vi "Actor Core.vi"(8 "error in":errorcluster, 11 "State in":refnum<class "Keypad.lvclass">) -> (0 "error out":errorcluster, 3 "Actor out":refnum<class "Actor.lvclass">)   [LabVIEW 2020, in "Keypad.lvlib" / "Keypad.lvclass"]
doc: "(<B>Filename</B>: Actor Framework.lvlib:Actor.lvclass:Actor Core.vi)\n\nThis override invokes Entry.vi on the initial state, prior to calling the parent Actor Core. Adding this behavior to Actor Core (instead of an override of Pre Launch Init.vi) allows the initial state to launch a nested actor as part of its entry behavior.\n\nReceives messages to the actor, reacts to them, and initiates any error handling that may shut the actor down.\n\nDescendant classes may override this VI to append parallel tasks for the actor to complete while it handles messages. Overrides use the Call Parent Method node."
uses:
  Keypad.lvclass
  <vilib>/ni/Actors/State Actor/State Actor/State Actor.lvclass
  <vilib>/ActorFramework/Actor/Actor.lvclass
  <vilib>/ActorFramework/Stop Msg/Stop Msg.lvclass
  Keypad Messages/Key Pressed Msg/Key Pressed Msg.lvclass
  Keypad Messages/Set NumLock Msg/Set NumLock Msg.lvclass
  Type Def - Entry Keypad Cluster.ctl
  Type Def - Cursor Display.ctl
panel:
  out "Locked?":bool
  in  "Num Lock":bool
  out "Cursor":T1
  in  "Keypad Cluster":T2
  out "Text":string
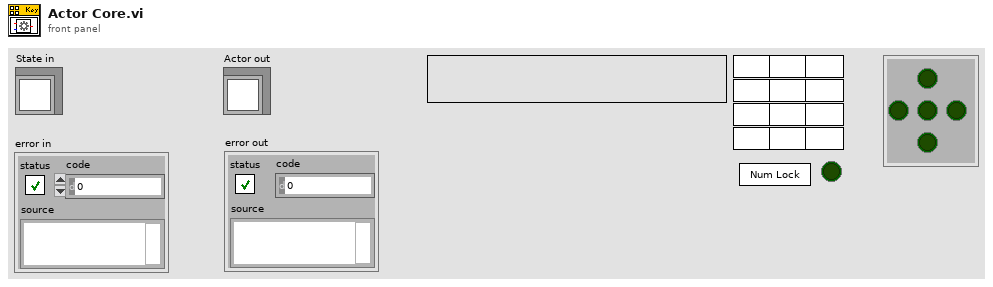
[diagram p1: front panel]
types:
  T1 = typedef "Type Def - Cursor Display.ctl" = cluster{"Up":bool, "Left":bool, "Ctr":bool, "Right":bool, "Down":bool}
  T2 = typedef "Type Def - Entry Keypad Cluster.ctl" = cluster{"K 0":bool, "K 1":bool, "K 2":bool, "K 3":bool, "K 4":bool, "K 5":bool, "K 6":bool, "K 7":bool, "K 8":bool, "K 9":bool, "K C":bool, "K E":bool}
  T3 = cluster{"Stop":refnum<user-event>, "Labels":refnum<user-event>, "Text":refnum<user-event>, "Cursor":refnum<user-event>, "NumLock":refnum<user-event>}
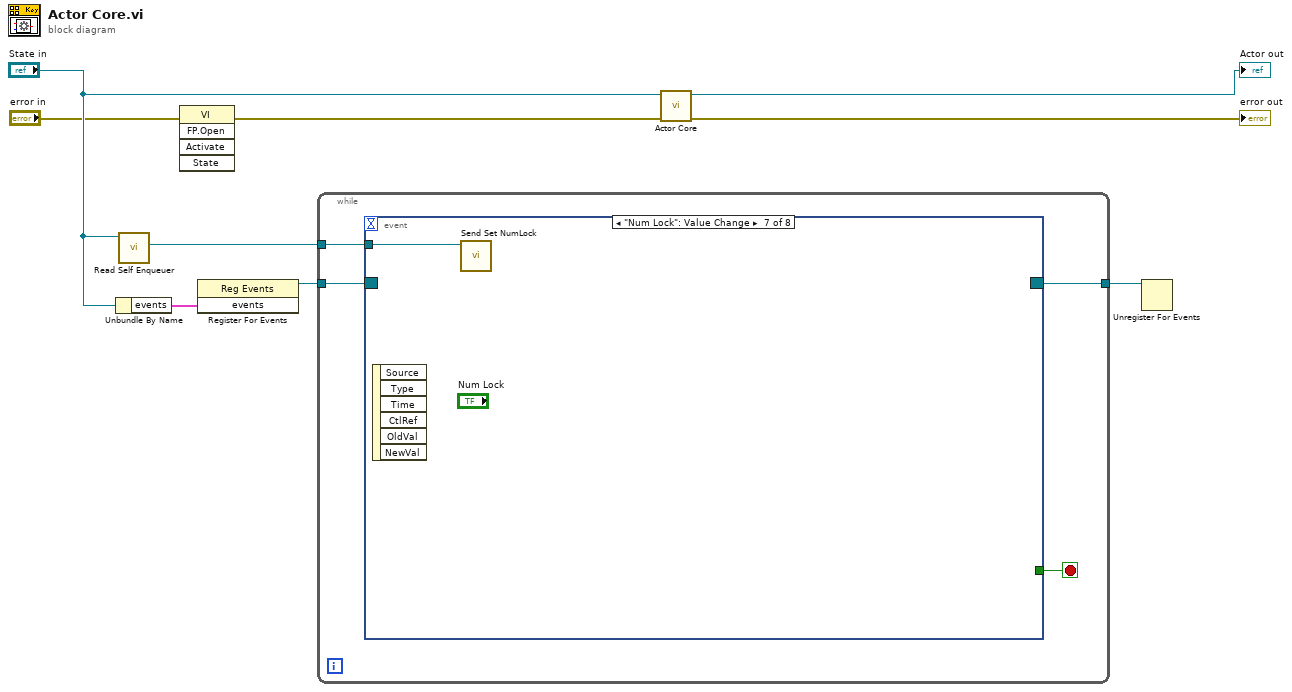
[diagram p0: block diagram]
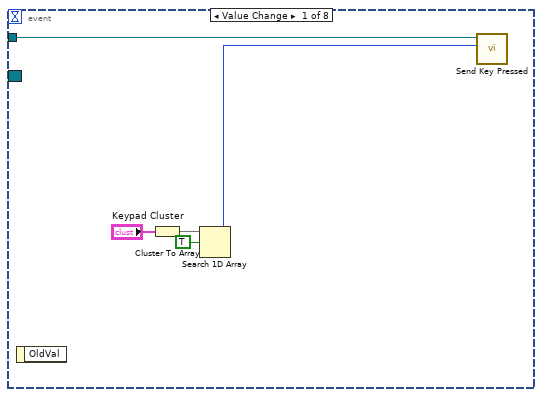
[diagram p2: hidden frame]
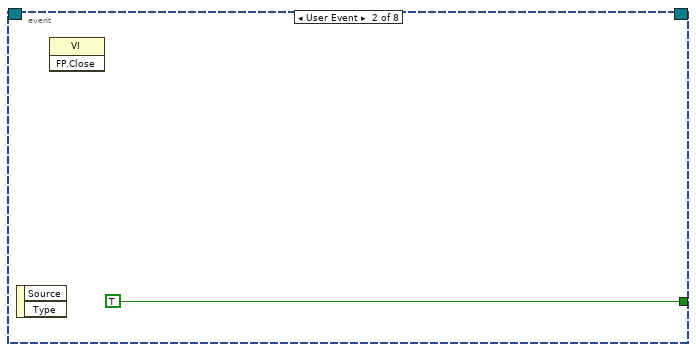
[diagram p3: hidden frame]
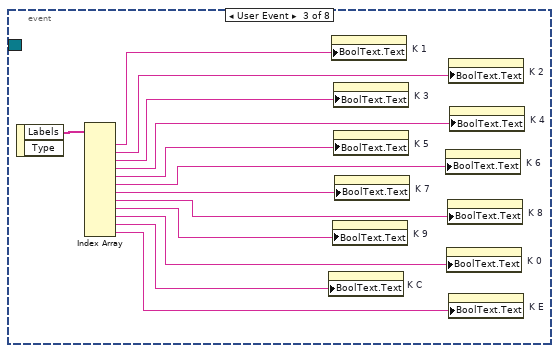
[diagram p4: hidden frame]
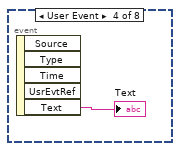
[diagram p5: hidden frame]
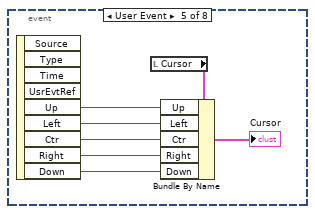
[diagram p6: hidden frame]
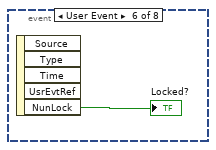
[diagram p7: hidden frame]
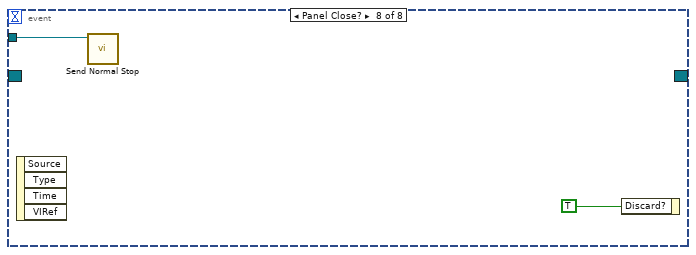
[diagram p8: hidden frame]
diagram:
  n1 = Unbundle By Name("State in") -> ("events"=w7:T3)
  n2 = call <vilib>:"Read Self Enqueuer.vi"("Actor"="State in") -> ("Self Enqueuer"=w4:refnum<class "Message Enqueuer.lvclass">)  [unwired: 10 in]
  n3 = invoke class="VI" method="FP.Open"(error in="error in") -> (error out=w2:errorcluster)  [unwired: 4 in, 4 out]
  n4 = register-events(w7) -> (reference out=w6:refnum<event-registration>)  [unwired: 2 in, 1 out]
  n5 = while {
    tunnel: w6 -> [w13]
    tunnel: w4 -> [w11]
    tunnel: [w10] -> w1
    stop <- w12 stop-if-true
    n6 = event shown="[6] \"Num Lock\": Value Change" {
      selector: w13 -> [_ _ _ _ _ _ _ _]
      dyn-events: [_ _ _ _ _ _ _ _] -> w10
      timeout: _ -> [_ _ _ _ _ _ _ _]
      tunnel: [_ TRUE _ _ _ _ _ _] -> w12
      tunnel: w11 -> [w15 _ _ _ _ _ w42 w43]
      event Value Change {
        n7 = event-data() -> ()  [unwired: 1 in, 1 out]
        n8 = Cluster To Array(cluster="Keypad Cluster") -> (array=w16:bool[])
        n9 = Search 1D Array(1D array=w16, element=TRUE) -> (index of element=w14:i32)  [unwired: 1 in]
        n10 = call "Send Key Pressed.vi"("Key Pressed"=w14, "Message Enqueuer"=w15) -> ()  [unwired: 8 in, 2 out]
      }
      event User Event {
        n11 = event-data() -> ()  [unwired: 1 in, 2 out]
        n12 = invoke class="VI" method="FP.Close"() -> ()  [unwired: 3 in, 3 out]
      }
      event User Event {
        n13 = event-data() -> ("Labels"=w32:string[])  [unwired: 1 in, 1 out]
        n14 = Index Array(array=w32) -> (element #1=w31:string, element #2=w30:string, element #3=w29:string, element #4=w28:string, element #5=w27:string, element #6=w26:string, element #7=w25:string, element #8=w24:string, element #9=w23:string, element #10=w22:string, element #11=w21:string, element #12=w20:string)  [unwired: 12 in]
        n15 = property on="K C" class="Bool"("BoolText.Text"=w21) -> ()  [unwired: 2 in, 2 out]
        n16 = property on="K 1" class="Bool"("BoolText.Text"=w31) -> ()  [unwired: 2 in, 2 out]
        n17 = property on="K 9" class="Bool"("BoolText.Text"=w23) -> ()  [unwired: 2 in, 2 out]
        n18 = property on="K 3" class="Bool"("BoolText.Text"=w29) -> ()  [unwired: 2 in, 2 out]
        n19 = property on="K 5" class="Bool"("BoolText.Text"=w27) -> ()  [unwired: 2 in, 2 out]
        n20 = property on="K 7" class="Bool"("BoolText.Text"=w25) -> ()  [unwired: 2 in, 2 out]
        n21 = property on="K 6" class="Bool"("BoolText.Text"=w26) -> ()  [unwired: 2 in, 2 out]
        n22 = property on="K 0" class="Bool"("BoolText.Text"=w22) -> ()  [unwired: 2 in, 2 out]
        n23 = property on="K 8" class="Bool"("BoolText.Text"=w24) -> ()  [unwired: 2 in, 2 out]
        n24 = property on="K 2" class="Bool"("BoolText.Text"=w30) -> ()  [unwired: 2 in, 2 out]
        n25 = property on="K E" class="Bool"("BoolText.Text"=w20) -> ()  [unwired: 2 in, 2 out]
        n26 = property on="K 4" class="Bool"("BoolText.Text"=w28) -> ()  [unwired: 2 in, 2 out]
      }
      event User Event {
        n27 = event-data() -> ("Text"=→"Text":string)  [unwired: 1 in, 4 out]
      }
      event User Event {
        n28 = event-data() -> ("Up"=w39:bool, "Left"=w38:bool, "Ctr"=w37:bool, "Right"=w36:bool, "Down"=w35:bool)  [unwired: 1 in, 4 out]
        n29 = local read "Cursor"() -> (w40:T1)
        n30 = Bundle By Name(cluster=w40, "Up"=w39, "Left"=w38, "Ctr"=w37, "Right"=w36, "Down"=w35) -> (→"Cursor":T1)
      }
      event User Event {
        n31 = event-data() -> ("NunLock"=→"Locked?":bool)  [unwired: 1 in, 4 out]
      }
      event "Num Lock": Value Change {
        n32 = event-data() -> ()  [unwired: 1 in, 6 out]
        n33 = call "Send Set NumLock.vi"("Message Enqueuer"=w42) -> ()  [unwired: 9 in, 2 out]
      }
      event Panel Close? {
        n34 = event-data() -> ()  [unwired: 1 in, 4 out]
        n35 = call <vilib>:"Send Normal Stop.vi"("Message Enqueuer"=w43) -> ()  [unwired: 10 in, 1 out]
        n36 = event-data("Discard?"=TRUE) -> ()  [unwired: 1 in, 1 out]
      }
    }
  }
  n37 = call-parent "Actor Core.vi"("error in"=w2, "State in"="State in") -> ("error out"=→"error out":errorcluster, "Actor out"=→"Actor out":refnum<class "Actor.lvclass">)  [unwired: 8 in]
  n38 = Unregister For Events(event registration refnum=w1) -> ()  [unwired: 1 in, 1 out]
